vi "Enqueue Prior.vi"(8 "Error In":errorcluster, 9 "Data":variant, 10 "State":string, 11 "Queue in":refnum<queue>) -> (0 "Error Out":errorcluster, 3 "Queue out":refnum<queue>)   [LabVIEW 2019, in "Queues.lvlib"]
uses:
  Message Cluster.ctl
  Queues.lvlib
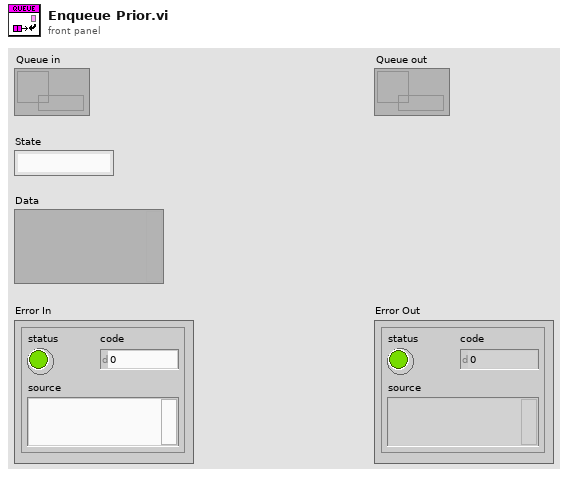
[diagram p1: front panel]
types:
  T1 = typedef "Queues.lvlib/Message Cluster.ctl" = cluster{"State":string, "Data":variant}
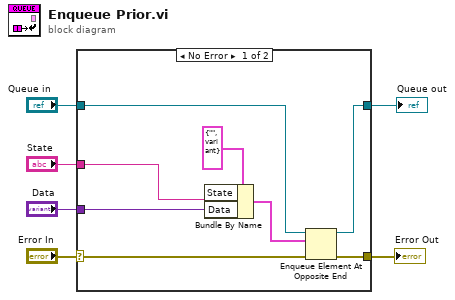
[diagram p0: block diagram]
diagram:
  n1 = case shown="No Error" "Error In" {
    selector: "Error In" -> [w9 w16]
    tunnel: "State" -> [w13 _]
    tunnel: "Data" -> [w12 _]
    tunnel: "Queue in" -> [w10 w15]
    tunnel: [w8 w16] -> w2
    tunnel: [w7 w15] -> w1
    frame No Error {
      n2 = Bundle By Name(cluster=T1 {"State"="", "Data"=variant} ("Message"), "State"=w13, "Data"=w12) -> (w11:T1)
      n3 = Enqueue Element At Opposite End(queue=w10, element=w11, error in (no error)=w9) -> (queue out=w7:refnum<queue>, error out=w8:errorcluster)  [unwired: 1 in, 1 out]
    }
    frame Error {
    }
  }
  "Error Out" <- w2
  "Queue out" <- w1
